vi "Client Configuration.vi"() -> ()   [LabVIEW 2013]
panel:
  in  "Host IP Address":string
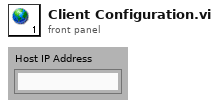
[diagram p1: front panel]
diagram:
